vi "Interface_Asset_Map Status.vi"(8 "error in (no error)":errorcluster, 11 "Interface_Asset in":refnum<class "Interface_Asset.lvclass">) -> (0 "error out":errorcluster, 3 "Interface_Asset out":refnum<class "Interface_Asset.lvclass">)   [LabVIEW 2015, in "Interface_Asset.lvclass"]
uses:
  Interface_Asset.lvclass
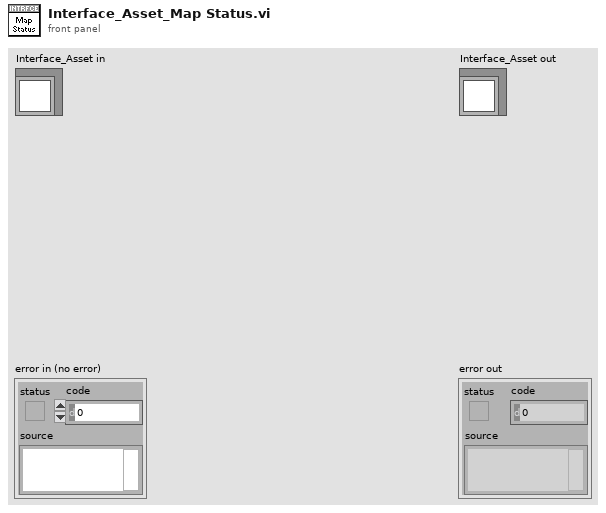
[diagram p1: front panel]
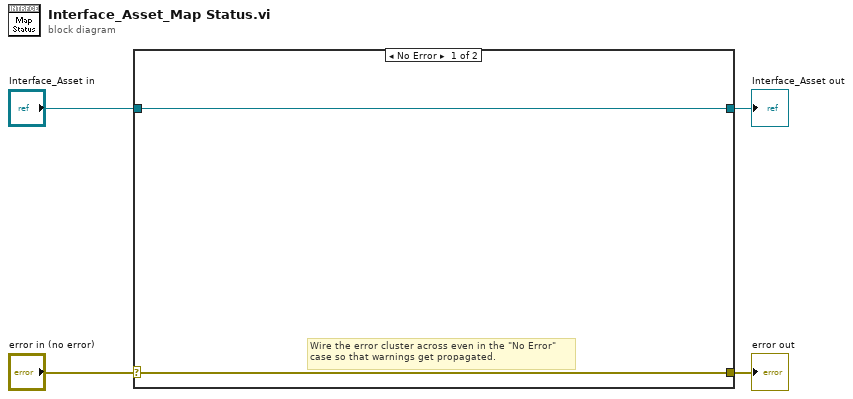
[diagram p0: block diagram]
diagram:
  n1 = case shown="No Error" "error in (no error)" {
    selector: "error in (no error)" -> [w5 w8]
    tunnel: [w5 w8] -> w3
    tunnel: [w6 w7] -> w1
    tunnel: "Interface_Asset in" -> [w6 w7]
    frame No Error {
      # "Wire the error cluster across even in the \"No Error\"\ncase so that warnings get propagated."
    }
    frame Error {
    }
  }
  "error out" <- w3
  "Interface_Asset out" <- w1
